vi "Packet decoder - GPS.vi"(8 "error in (no error)":errorcluster, 10 "Packet array":u8[](array[numeric]), 11 "Input packet":T1) -> (0 "error out":errorcluster, 2 "Valid packet":bool, 3 "Output packet":T1)   [LabVIEW 2015, in "Acquisition.lvlib"]
uses:
  Acquisition.lvlib
  Generic data packet.ctl
  My Graphs/Gps Map Graph coordinates.ctl
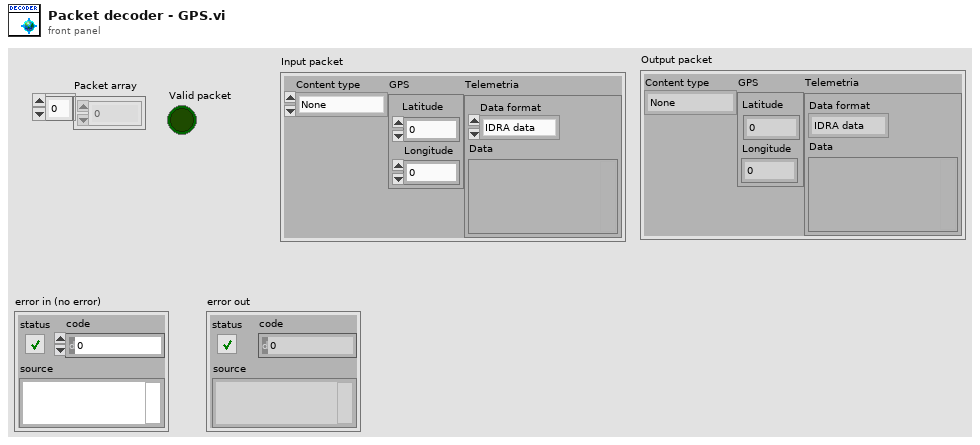
[diagram p1: front panel]
types:
  T1 = typedef "Acquisition.lvlib/Generic data packet.ctl" = cluster{"Content type":enum16{"None", "Telemetria", "GPS"}, "GPS":T2, "Telemetria":cluster{"Data format":enum16{"IDRA data", "XAM data"}, "Data":variant}}
  T2 = typedef "Gps Map Graph coordinates.ctl" = cluster{"Latitude":dbl, "Longitude":dbl}
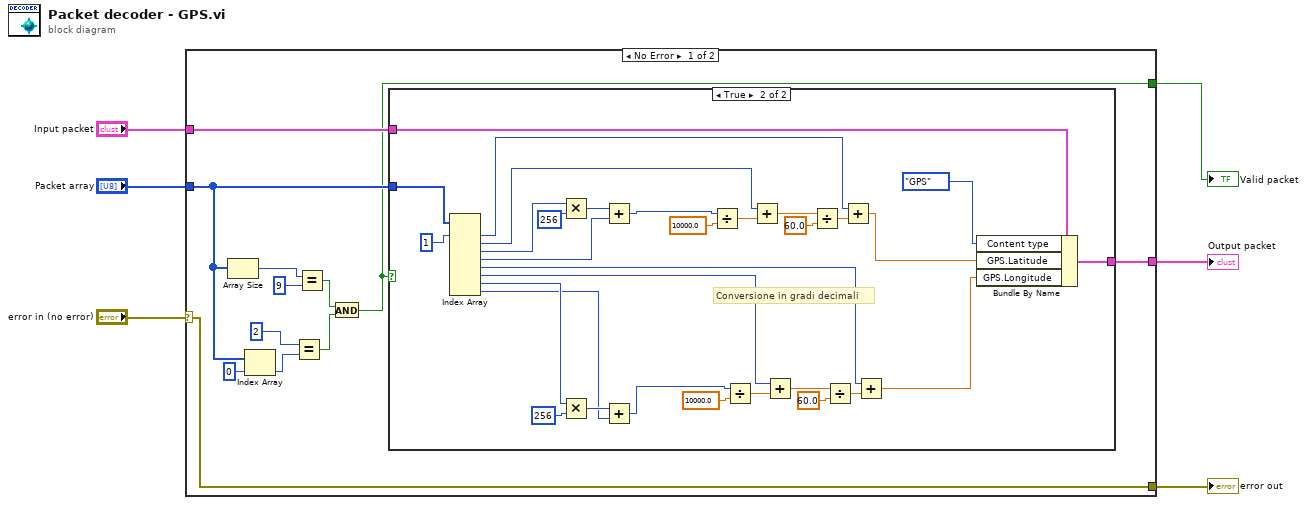
[diagram p0: block diagram]
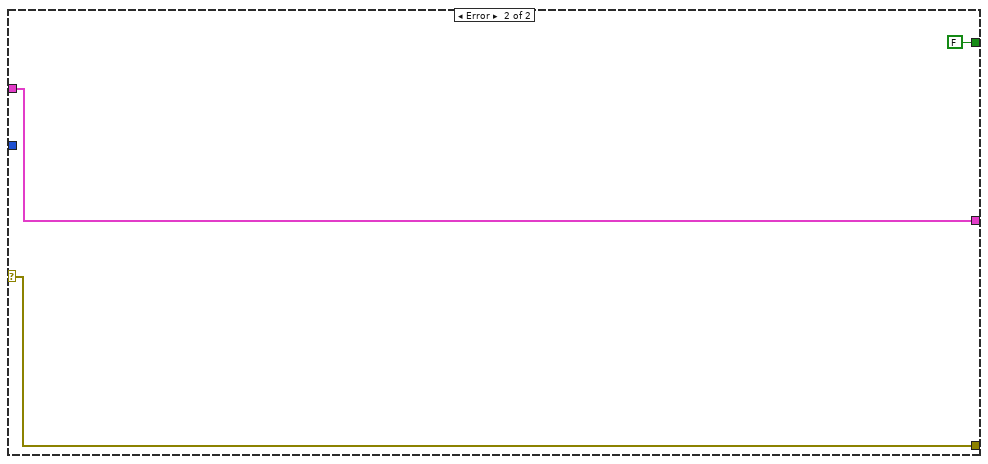
[diagram p3: hidden frame]
diagram:
  n1 = case shown="No Error" "error in (no error)" {
    selector: "error in (no error)" -> [w18 w53]
    tunnel: [w18 w53] -> w5
    tunnel: "Packet array" -> [w17 _]
    tunnel: [w9 w52] -> w2
    tunnel: "Input packet" -> [w8 w52]
    tunnel: [w7 FALSE] -> w1
    frame No Error {
      n2 = Array Size(array=w17) -> (size(s)=w12:i32)
      n3 = Index Array(array=w17, index=0) -> (element=w15:u8)
      n4 = Equal?(x=u8 2, y=w15) -> (x = y?=w13:bool)
      n5 = Equal?(x=w12, y=9) -> (x = y?=w14:bool)
      n6 = And(x=w14, y=w13) -> (x .and. y?=w7:bool)
      n7 = case shown="True" w7 {
        tunnel: w17 -> [_ w45]
        tunnel: [w19 w30] -> w9
        tunnel: w8 -> [w19 w31]
        frame False {
        }
        frame True {
          # "Conversione in gradi decimali"
          n8 = Index Array(array=w45, index #1=1 ("index")) -> (element #1=w34:u8, element #2=w26:u8, element #3=w25:u8, element #4=w24:u8, element #5=w23:u8, element #6=w22:u8, element #7=w21:u8, element #8=w20:u8)  [unwired: 7 in]
          n9 = Multiply(x=w25, y=u16 256) -> (x*y=w50:u16)
          n10 = Multiply(x=w21, y=u16 256) -> (x*y=w47:u16)
          n11 = Add(x=w50, y=w24) -> (x+y=w33:u16)
          n12 = Add(x=w47, y=w20) -> (x+y=w32:u16)
          n13 = Divide(x=w33, y=10000.0) -> (x/y=w43:dbl)
          n14 = Divide(x=w32, y=10000.0) -> (x/y=w36:dbl)
          n15 = Add(x=w26, y=w43) -> (x+y=w42:dbl)
          n16 = Add(x=w22, y=w36) -> (x+y=w37:dbl)
          n17 = Divide(x=w42, y=60.0) -> (x/y=w44:dbl)
          n18 = Divide(x=w37, y=60.0) -> (x/y=w35:dbl)
          n19 = Add(x=w34, y=w44) -> (x+y=w28:dbl)
          n20 = Add(x=w23, y=w35) -> (x+y=w27:dbl)
          n21 = Bundle By Name(cluster=w31, "Content type"=enum16{"None", "Telemetria", "GPS"}."GPS", "GPS.Latitude"=w28, "GPS.Longitude"=w27) -> (w30:T1)
        }
      }
    }
    frame Error {
    }
  }
  "error out" <- w5
  "Valid packet" <- w1
  "Output packet" <- w2
